vi "peak -- find -- pm - V1 - test.vi"(0 "omega in":dbl[](array[numeric]), 1 "z in":cdb[](array[numeric]), 3 "cursor window":T7={"left"=2378.60310421286, "right "=2421.6740576496672, "center"=2421.6740576496672, "window"=2421.6740576496672, "cursors"=[], "relative"=0, "absolute"=0, "fixed vertical offset"=2421.6740576496672, "vertical offset"=2421.6740576496672, "skew"=2421.6740576496672, "default window frac"=2421.6740576496672, "kind"=enum."fancy", "skew.left"=2421.6740576496672, "skew.right"=0.0, "Plot ref"=refnum, "wing order"=enum."back"}, 5 "parameters: complex fit":T4={"main VI path"=path "", "scale factor"=3.0, "# of grid points"=200, "parameters: wavepacket"={"R"=0.5, "wave number"=22.0, "delta k"=7.0, "radii vector"=[], "radial section"=[], "wave vector"=22.0, "wavepacket is"=TRUE}, "span"=0.27789, "interference ?"=enum."cp z center", "filter method"=enum."three"} {"span" min=0.0 max=0.5 step=1e-05 scale=0.0001..0.5 scale format="%#_5f"; "parameters: wavepacket"."delta k" format="%#_3f"; "parameters: wavepacket"."wave number" format="%#_3f"; "parameters: wavepacket"."R" format="%#_3f"}, 6 "plot what":enum16{"plot pm", "plot cp", "a"}(ring), 7 "plots: filter related":T3, 8 "plot staff":enum16{"plot", "do not plot", "a"}(ring)) -> (14 "# points in window":dbl, 17 "good lorentzian":T1={"Amplitude"=-1.0311345636926572, "omega(0)"=-1.0311345636926572, "Gamma"=-1.0311345636926572, "phase"=-1.0311345636926572, "Q"=-1.0311345636926572, "Norm  Ampl"=-1.0311345636926572, "z (inf)"=-1.0311345636926572+0.0i, "4corners"={"z (-pi/2)"=-1.0311345636926572+0.5736824521422934i, "z(inf)"=-0.5200164984937075+1.0975277942502903i, "z (pi/2)"=-1.0311345636926572+0.5736824521422934i, "z center"=-0.5136528600391839+0.580046090596817i, "z(0)"=-0.5200164984937075+1.0975277942502903i, "radius"=-1.0311345636926572}} {"z (inf)" format="%#9_9f"; "Q" format="%#9_9f"; "phase" format="%#9_9f"; "Gamma" format="%#9_9f"; "omega(0)" format="%#9_9f"}, 18 "pm lorentzian":T1={"Amplitude"=-1.0311345636926572, "omega(0)"=-1.0311345636926572, "Gamma"=-1.0311345636926572, "phase"=-1.0311345636926572, "Q"=-1.0311345636926572, "Norm  Ampl"=-1.0311345636926572, "z (inf)"=-1.0311345636926572+0.0i, "4corners"={"z (-pi/2)"=-1.0311345636926572+0.5736824521422934i, "z(inf)"=-0.5200164984937075+1.0975277942502903i, "z (pi/2)"=-1.0311345636926572+0.5736824521422934i, "z center"=-0.5136528600391839+0.580046090596817i, "z(0)"=-0.5200164984937075+1.0975277942502903i, "radius"=-1.0311345636926572}} {"z (inf)" format="%#9_9f"; "Q" format="%#9_9f"; "phase" format="%#9_9f"; "Gamma" format="%#9_9f"; "omega(0)" format="%#9_9f"}, 19 "cp lorentzian":T1={"Amplitude"=-1.0311345636926572, "omega(0)"=-1.0311345636926572, "Gamma"=-1.0311345636926572, "phase"=-1.0311345636926572, "Q"=-1.0311345636926572, "Norm  Ampl"=-1.0311345636926572, "z (inf)"=-1.0311345636926572+0.0i, "4corners"={"z (-pi/2)"=-1.0311345636926572+0.5736824521422934i, "z(inf)"=-0.5200164984937075+1.0975277942502903i, "z (pi/2)"=-1.0311345636926572+0.5736824521422934i, "z center"=-0.5136528600391839+0.580046090596817i, "z(0)"=-0.5200164984937075+1.0975277942502903i, "radius"=-1.0311345636926572}} {"z (inf)" format="%#9_9f"; "Q" format="%#9_9f"; "phase" format="%#9_9f"; "Gamma" format="%#9_9f"; "omega(0)" format="%#9_9f"})   [LabVIEW 2012]
uses:
  filter method control.ctl
  cursor winow.ctl
  lorentzian.ctl
  circle corners.ctl
  peak -- parameters -- complex fit.ctl
  wavepacket.ctl
  plot refs -- filter related.ctl
  tale of three indices.vi
  Q -- check range -- i -- real.vi
  filter -- window span logic.vi
  linear interp iiii- complex - z-omega - divide.vi
  linear interpolation iiii- complex.vi
  containing bix.vi
  peak -- guess at omega -- dzdomega.vi
  command stack.vi
  tale of three indices -- check state.vi
  Q -- check range -- i -- integer.vi
  Q - not nan -- real.vi
  linear interp iiii- complex - z-omega.vi
  line -- complex.vi
  peak -- z center from mult phase points.vi
  peak -- four corner circle transformation logic.vi
  peak - fit phase around center - V1.vi
  peak -- estimate for lorentzian.vi
  peak -- fake phase around center.vi
  peak -- get weights.vi
  Q - not nan -- integer.vi
  circle center from three points.vi
  <vilib>/Analysis/baseanly.llb/A x B.vi
  <vilib>/Analysis/baseanly.llb/Complex A x B.vi
  <vilib>/Analysis/baseanly.llb/Inverse Matrix.vi
  <vilib>/Analysis/baseanly.llb/Real Inverse Matrix.vi
  <vilib>/Analysis/Matrix/Numeric/Conversions/Array To Matrix.vi
  <vilib>/Analysis/Matrix/Numeric/Conversions/Array To Matrix - RA2.vi
  array - generate range.vi
  <vilib>/Utility/error.llb/Clear Errors.vi
  <vilib>/gmath/NumericalOptimization/Nonlinear Curve Fit.vi
  <vilib>/gmath/NumericalOptimization/Nonlinear Curve Fit LM.vi
  peak -- fit function -- arctan.vi
panel:
  in  "span":dbl=0.01
  in  "filter method":T6=enum."three"
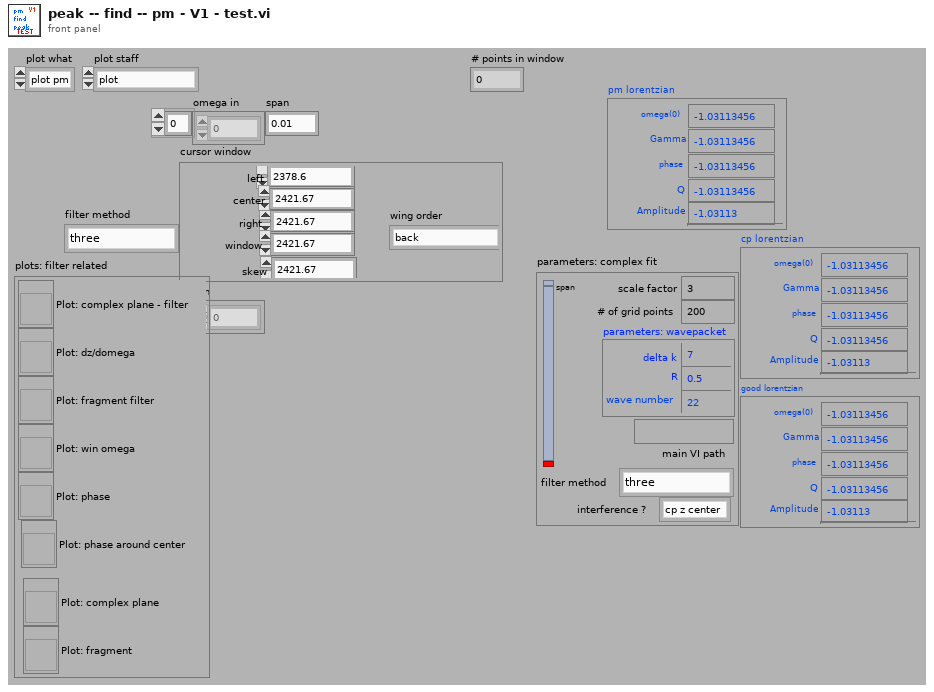
[diagram p1: front panel]
types:
  T1 = typedef "lorentzian.ctl" = cluster{"Amplitude":dbl, "omega(0)":dbl, "Gamma":dbl, "phase":dbl, "Q":dbl, "Norm  Ampl":dbl, "z (inf)":cdb, "4corners":T2}
  T2 = typedef "circle corners.ctl" = cluster{"z (-pi/2)":cdb, "z(inf)":cdb, "z (pi/2)":cdb, "z center":cdb, "z(0)":cdb, "radius":dbl}
  T3 = typedef "plot refs -- filter related.ctl" = cluster{"Plot: complex plane - filter":refnum<vi>, "Plot: dz/domega":refnum<vi>, "Plot: fragment filter":refnum<vi>, "Plot: win omega":refnum<vi>, "Plot: phase":refnum<vi>, "Plot: phase around center":refnum<vi>, "Plot: complex plane":refnum<vi>, "Plot: fragment":refnum<vi>}
  T4 = typedef "peak -- parameters -- complex fit.ctl" = cluster{"main VI path":path, "scale factor":dbl, "# of grid points":i32, "parameters: wavepacket":T5, "span":dbl, "interference ?":enum16{"cp z center", "pm zcenter", "fancy"}, "filter method":T6}
  T5 = typedef "wavepacket.ctl" = cluster{"R":dbl, "wave number":dbl, "delta k":dbl, "radii vector":dbl[], "radial section":cdb[], "wave vector":dbl, "wavepacket is":bool}
  T6 = typedef "filter method control.ctl" = enum16{"four", "five", "one", "two", "three", "zero", "minus one", "minus two"}
  T7 = typedef "cursor winow.ctl" = cluster{"left":dbl, "right ":dbl, "center":dbl, "window":dbl, "cursors":i32[], "relative":i32, "absolute":i32, "fixed vertical offset":dbl, "vertical offset":dbl, "skew":dbl, "default window frac":dbl, "kind":enum16{"symmetric", "skewed", "fancy"}, "skew.left":dbl, "skew.right":dbl, "Plot ref":refnum<vi>, "wing order":enum16{"forw", "back"}}
  T8 = typedef "tale of three indices -- int -- control.ctl" = cluster{"left":i32, "center":i32, "right":i32, "right most":i32, "left most":i32, "window":i32, "max win factor":i32, "max win":i32, "min win":i32}
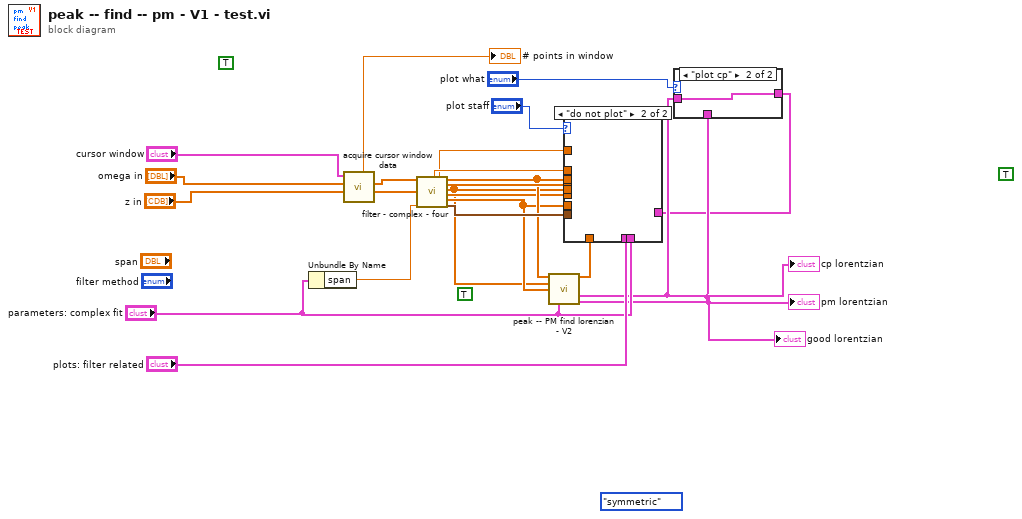
[diagram p0: block diagram]
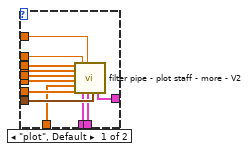
[diagram p2: hidden frame]
diagram:
  (unwired) TRUE
  (unwired) TRUE
  (unwired) enum16{"symmetric", "skewed", "fancy"}."symmetric" ("kind")
  (unwired) TRUE
  n1 = Unbundle By Name("parameters: complex fit") -> ("span"=w5:dbl)
  n2 = call "acquire cursor window data.vi"("z in"="z in", "omega in"="omega in", "cursor window"="cursor window") -> ("z out"=w7:cdb[], "omega  out"=w8:dbl[], "length index"=→"# points in window":dbl)  [unwired: 4 in, 2 out]
  n3 = call "filter - complex - four.vi"("omega  in"=w8, "z in"=w7, "span"=w5) -> ("center"=w13:cdb, "norm"=w12:dbl, "omega out"=w14:dbl[], "z in out"=w15:cdb[], "z out"=w6:cdb[], "win omega out"=w11:dbl[], "dz/domega out"=w10:cdb[], "tale of three"=w16:T8)  [unwired: 9 in]
  n4 = call "peak -- PM find lorenzian - V2.vi"("omega"=w14, "z"=w6, "dz/domega"=w10, "parameters: complex fit"="parameters: complex fit") -> ("phase (around center)"=w9:dbl[], "cp lorentzian"=w18:T1, "poor man lorentzian"=w17:T1)  [unwired: 8 in, 1 out]
  "pm lorentzian" <- w17
  "cp lorentzian" <- w18
  "good lorentzian" <- w17
  n5 = case shown="\"plot cp\"" "plot what" {
    tunnel: [w24 w25] -> w3
    tunnel: w18 -> [_ w25]
    tunnel: w17 -> [w24 _]
    frame "plot pm", Default {
    }
    frame "plot cp" {
    }
  }
  n6 = case shown="\"do not plot\"" "plot staff" {
    tunnel: w16 -> [w37 _]
    tunnel: w15 -> [w36 _]
    tunnel: w14 -> [w35 _]
    tunnel: w13 -> [w34 _]
    tunnel: w12 -> [w33 _]
    tunnel: w11 -> [w32 _]
    tunnel: w10 -> [w31 _]
    tunnel: w9 -> [w30 _]
    tunnel: w6 -> [w29 _]
    tunnel: "plots: filter related" -> [w28 _]
    tunnel: "parameters: complex fit" -> [w27 _]
    tunnel: w3 -> [w26 _]
    frame "plot", Default {
      n7 = call "filter pipe - plot staff - more - V2.vi"("omega  in"=w35, "zin"=w36, "z out"=w29, "win omega"=w32, "phase"=w30, "dz/domega in"=w31, "center"=w34, "plots: filter related"=w28, "norm"=w33, "parameters: complex fit"=w27, "tale of three indices -- int -- control"=w37, "lorentzian"=w26) -> ()  [unwired: 8 in]
    }
    frame "do not plot" {
    }
  }
